vi "Read Inputs from system.vi"(8 "error in":errorcluster, 11 "System Diagnostics runtime in":refnum<class "System Diagnostics runtime.lvclass">) -> (0 "error out":errorcluster, 2 "Inputs from system":T1, 3 "System Diagnostics runtime out":refnum<class "System Diagnostics runtime.lvclass">)   [LabVIEW 2013, in "System Diagnostics runtime.lvclass"]
uses:
  System Diagnostics runtime.lvclass
  configuration/input data indices.ctl
  System Diagnostics runtime.lvclass/System Diagnostics runtime.ctl
  configuration/System Diagnostics configuration.lvclass
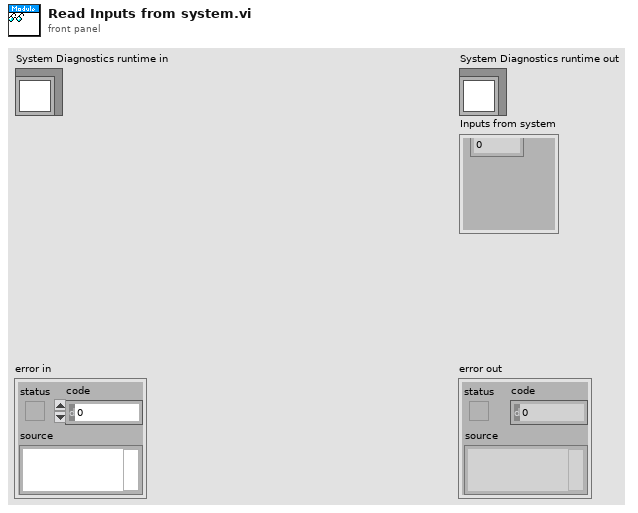
[diagram p1: front panel]
types:
  T1 = typedef "System Diagnostics configuration.lvclass/input data indices.ctl" = cluster{"Double.CPU load average":i32, "Double.timed structures load":i32, "Double.free memory":i32, "Double.contiguous memory":i32}
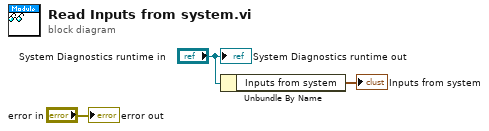
[diagram p0: block diagram]
diagram:
  n1 = Unbundle By Name("System Diagnostics runtime in") -> ("Inputs from system"=→"Inputs from system":T1)
  "error out" <- "error in"
  "System Diagnostics runtime out" <- "System Diagnostics runtime in"
